vi "PicoScope4000aSetDataBuffers.vi"(5 "enabled array":i16[](array[numeric]), 7 "Buffer and Transfer Settings":T2={"startIndex"=0, "Samples"=1000, "Down Sample Ratio"=1, "Down-Sample Mode"=1} {"Down-Sample Mode" items=["RAW none"=2147483648, "None"=0, "Aggregate"=1, "Decimate"=2, "Average"=4]; "Down Sample Ratio" step=1; "Samples" format="%_6p"}, 8 "error in (no error)":errorcluster, 10 "Data Pointers In":T1, 11 "handle in":i16) -> (0 "error out":errorcluster, 3 "handle out":i16)   [LabVIEW 2010]
doc: "Calls SetDataBuffers, and assigns Pico buffers"
uses:
  ps4000a.dll
  shared/PicoBuffers.ctl
  shared/Buffer and Transfer Settings.ctl
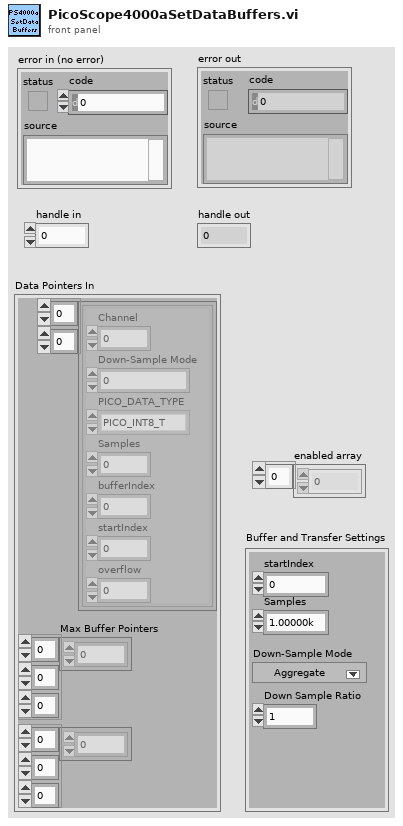
[diagram p1: front panel]
types:
  T1 = typedef "PicoBuffers.ctl" = cluster{"Max Buffer Pointers":u64[][][], "Min Buffer Pointers":u64[][][], "StreamingDataInfo":cluster{"Channel":u32, "Down-Sample Mode":u32, "PICO_DATA_TYPE":enum32{"PICO_INT8_T", "PICO_INT16_T", "PICO_INT32_T", "PICO_UINT32_T", "PICO_INT64_T", ""}, "Samples":i32, "bufferIndex":u64, "startIndex":i32, "overflow":i16}[][]}
  T2 = typedef "Buffer and Transfer Settings.ctl" = cluster{"startIndex":u64, "Samples":u64, "Down Sample Ratio":u64, "Down-Sample Mode":u32}
  T3 = cluster{"status":bool, "code":u32, "source":string}
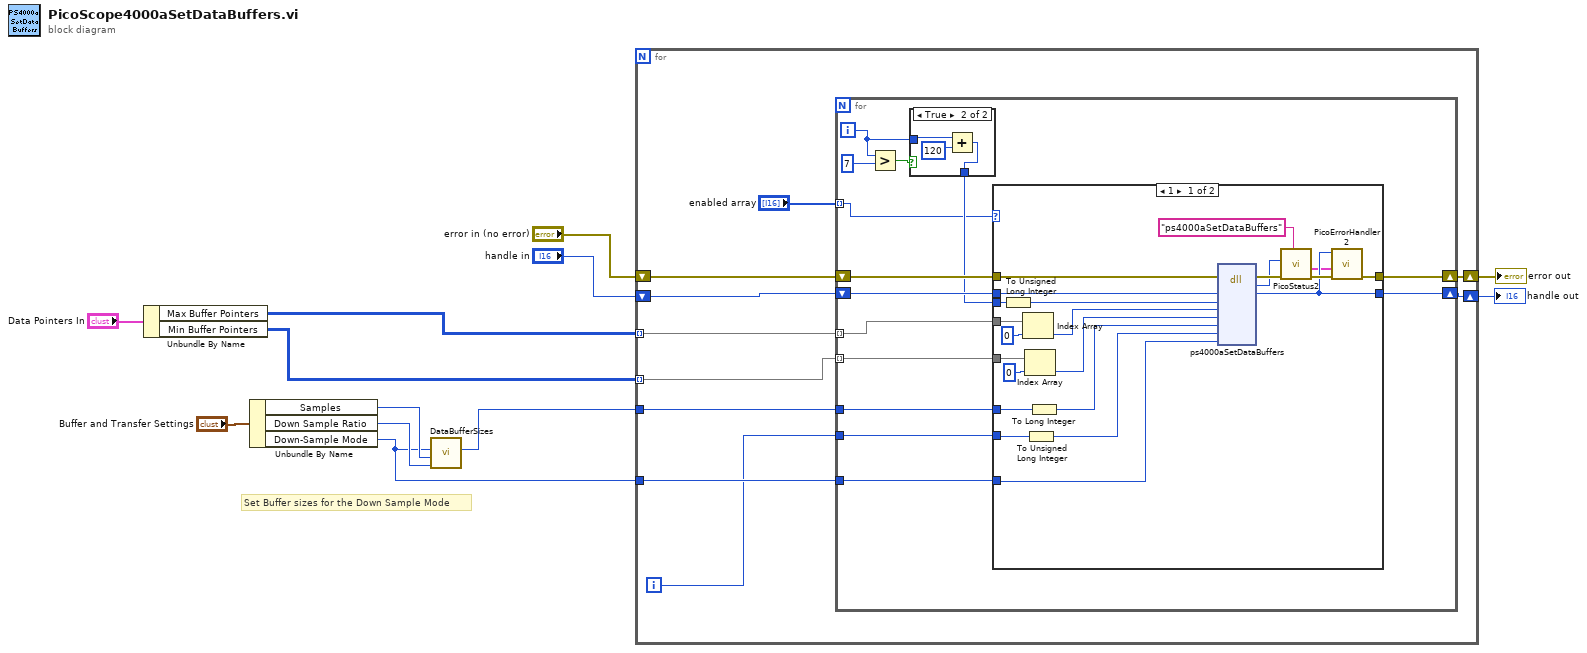
[diagram p0: block diagram]
diagram:
  # "Set Buffer sizes for the Down Sample Mode"
  n1 = Unbundle By Name("Data Pointers In") -> ("Max Buffer Pointers"=w2:u64[][][], "Min Buffer Pointers"=w1:u64[][][])
  n2 = Unbundle By Name("Buffer and Transfer Settings") -> ("Samples"=w4:u64, "Down Sample Ratio"=w5:u64, "Down-Sample Mode"=w3:u32)
  n3 = call "DataBufferSizes.vi"("Down Sample Ratio"=w5, "Number of Samples"=w4, "Down-Sample Mode"=w3) -> ("Max Buffer Size"=w6:i32)  [unwired: 7 in, 1 out]
  n4 = for {
    tunnel: w6 -> [w18]
    tunnel: w3 -> [w17]
    tunnel: w2 -> [w16] mode=indexing
    tunnel: w1 -> [w15] mode=indexing
    shift-right: [w22] -> w11
    shift-left: "error in (no error)" -> [w20]
    shift-right: [w21] -> w10
    shift-left: "handle in" -> [w19]
    i -> [w13]
    n5 = for {
      tunnel: w17 -> [w36]
      tunnel: w18 -> [w30]
      tunnel: "enabled array" -> [w23] mode=indexing
      tunnel: w16 -> [w29] mode=indexing
      shift-right: [w28] -> w22
      shift-left: w20 -> [w35]
      tunnel: w15 -> [w26] mode=indexing
      shift-right: [w25] -> w21
      shift-left: w19 -> [w34]
      tunnel: w13 -> [w24]
      i -> [w27]
      n6 = Greater?(x=w27, y=7) -> (0:w32:bool)
      n7 = case shown="True" w32 {
        tunnel: [w61 w62] -> w31
        tunnel: w27 -> [w61 w64]
        frame False {
        }
        frame True {
          n8 = Add(x=w64, y=120) -> (x+y=w62:i32)
        }
      }
      n9 = case shown="1" w23 {
        tunnel: w31 -> [w48 _]
        tunnel: w35 -> [w58 w60]
        tunnel: w34 -> [w55 w59]
        tunnel: w36 -> [w40 _]
        tunnel: [w52 w60] -> w28
        tunnel: [w51 w59] -> w25
        tunnel: w30 -> [w50 _]
        tunnel: w29 -> [w44 _]
        tunnel: w26 -> [w41 _]
        tunnel: w24 -> [w39 _]
        frame 1 {
          n10 = To Unsigned Long Integer(number=w48) -> (unsigned 32bit integer=w47:u32)
          n11 = Index Array(array=w44, index=0) -> (element=w45:u64)
          n12 = Index Array(array=w41, index=0) -> (element=w42:u64)
          n13 = To Unsigned Long Integer(number=w39) -> (unsigned 32bit integer=w38:u32)
          n14 = To Long Integer(number=w50) -> (32bit integer=w49:i32)
          n15 = dll-call lib="ps4000a.dll" fn="ps4000aSetDataBuffers" ("ps3000.dll:_ps3000_open_unit@0")(error in=w58, "handle"=w55, "channel"=w47, "bufferMax"=w45, "bufferMin"=w42, "bufferLth"=w49, "segmentIndex"=w38, "downSampleRatioMode"=w40) -> (error out=w57:errorcluster, "PICO_STATUS"=w56:u32, "handle"=w51:i16)  [unwired: 8 in, 1 out]
          n16 = call "PicoStatus2.vi"("PICO source"="ps4000aSetDataBuffers" ("source"), "Error in"=w57, "PICO STATUS"=w56) -> ("error out"=w53:errorcluster, "PICO_STATUS out"=w37:T3)  [unwired: 5 in]
          n17 = call "PicoErrorHandler2.vi"("error in (no error)"=w53, "PICO_STATUS in"=w37, "handle In"=w51) -> ("error out"=w52:errorcluster)  [unwired: 8 in]
        }
        frame 0, Default {
        }
      }
    }
  }
  "error out" <- w11
  "handle out" <- w10
